vi "Duplicate State.vi"(5 "Category to Duplicate (optional)":string, 6 "Before? (F: After)":bool, 7 "State to Duplicate":string, 8 "error in (no error)":errorcluster, 9 "New State":string, 10 "New Category (\"\": Use Existing)":string, 11 "JKI SM in":refnum<class "JKI SM.lvclass">) -> (0 "error out":errorcluster, 3 "JKI SM out":refnum<class "JKI SM.lvclass">)   [LabVIEW 2020, in "JKI State Machine API.lvlib" / "JKI SM.lvclass"]
uses:
  JKI SM.lvclass
  JKI SM.lvclass/JKI SM.ctl
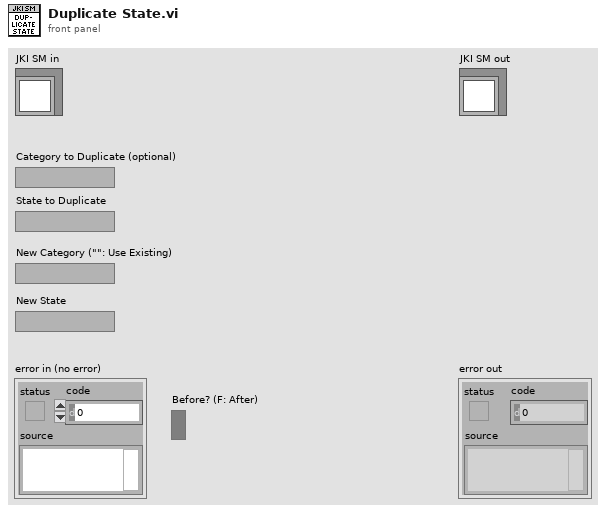
[diagram p1: front panel]
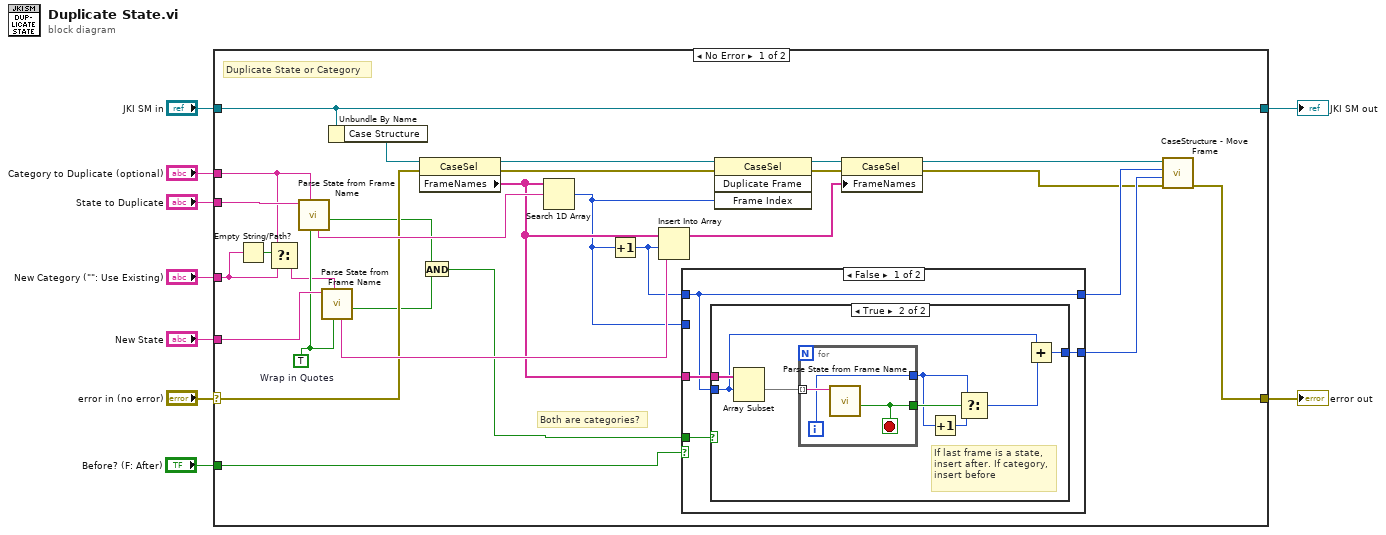
[diagram p0: block diagram]
diagram:
  n1 = case shown="No Error" "error in (no error)" {
    selector: "error in (no error)" -> [w23 w58]
    tunnel: [w22 w58] -> w8
    tunnel: [w31 w57] -> w6
    tunnel: "JKI SM in" -> [w31 w57]
    tunnel: "Category to Duplicate (optional)" -> [w34 _]
    tunnel: "State to Duplicate" -> [w38 _]
    tunnel: "New Category (\"\": Use Existing)" -> [w33 _]
    tunnel: "New State" -> [w37 _]
    tunnel: "Before? (F: After)" -> [w15 _]
    frame No Error {
      w36 = TRUE  # Wrap in Quotes
      # "Both are categories?"
      # "Duplicate State or Category"
      n2 = Empty String/Path?(string/path=w33) -> (empty?=w35:bool)
      n3 = Select(t=w34, s=w35, f=w33) -> (s? t:f=w32:string)
      n4 = call "Parse State from Frame Name.vi"("Wrap in Quotes? (FALSE)"=w36, "Category (Optional)"=w34, "Frame or State Name"=w38) -> ("is a Category Frame?"=w20:bool, "\"Category: State\" String"=w29:string)  [unwired: 3 in, 4 out]
      n5 = call "Parse State from Frame Name.vi"("Wrap in Quotes? (FALSE)"=w36, "Category (Optional)"=w32, "Frame or State Name"=w37) -> ("is a Category Frame?"=w19:bool, "\"Category: State\" String"=w27:string)  [unwired: 3 in, 4 out]
      n6 = Unbundle By Name(w31) -> ("Case Structure"=w30:refnum<vi>)
      n7 = property class="CaseSel"(reference=w30, error in=w23) -> (reference out=w28:refnum<vi>, error out=w24:errorcluster, "FrameNames"=w21:string[])
      n8 = And(x=w20, y=w19) -> (x .and. y?=w16:bool)
      n9 = Search 1D Array(1D array=w21, element=w29) -> (index of element=w12:i32)  [unwired: 1 in]
      n10 = Increment(x=w12) -> (x+1=w13:i32)
      n11 = Insert Into Array(array=w21, index=w13, new element=w27) -> (w18:string[])
      n12 = case shown="False" w15 {
        tunnel: w21 -> [w42 _]
        tunnel: [w41 w55] -> w17
        tunnel: w13 -> [w39 w55]
        tunnel: w16 -> [w40 _]
        tunnel: [w39 w56] -> w14
        tunnel: w12 -> [_ w56]
        frame False {
          n13 = case shown="True" w40 {
            tunnel: w42 -> [_ w50]
            tunnel: [w43 w49] -> w41
            tunnel: w39 -> [w43 w48]
            frame False {
            }
            frame True {
              # "If last frame is a state,\ninsert after. If category,\ninsert before"
              n14 = Array Subset(array=w50, index=w48) -> (w51:string[])  [unwired: 1 in]
              n15 = for {
                tunnel: w51 -> [w54] mode=indexing
                tunnel: [w53] -> w45
                tunnel: [w52] -> w47
                i -> [w53]
                stop <- w52 stop-if-true
                n16 = call "Parse State from Frame Name.vi"("Frame or State Name"=w54) -> ("is a Category Frame?"=w52:bool)  [unwired: 5 in, 5 out]
              }
              n17 = Increment(x=w45) -> (x+1=w44:i32)
              n18 = Select(t=w45, s=w47, f=w44) -> (s? t:f=w46:i32)
              n19 = Add(x=w48, y=w46) -> (x+y=w49:i32)
            }
          }
        }
        frame True {
        }
      }
      n20 = invoke class="CaseSel" method="Duplicate Frame"(reference=w28, error in=w24, "Frame Index"=w12) -> (reference out=w26:refnum<vi>, error out=w25:errorcluster)  [unwired: 1 in, 2 out]
      n21 = property class="CaseSel"(reference=w26, error in=w25, "FrameNames"=w18) -> (reference out=w11:refnum<vi>, error out=w10:errorcluster)
      n22 = call "CaseStructure - Move Frame.vi"("error in (no error)"=w10, "New Position"=w17, "Current Position"=w14, "CaseStructure in"=w11) -> ("error out"=w22:errorcluster)  [unwired: 6 in, 1 out]
    }
    frame Error {
    }
  }
  "error out" <- w8
  "JKI SM out" <- w6
